vi "Read Data From run Files.vi"(0 "Rack":i8, 1 "Rack Position":i8, 2 ".run File Path":path=path "\\\\beco\\autoage/runs/pos", 3 "System Number":string) -> (4 "Serial Number":string, 5 "Unit Type":string, 6 "Customer":string, 7 "Nominal Frequency":string, 8 "Gate Time":string)   [LabVIEW 2021]
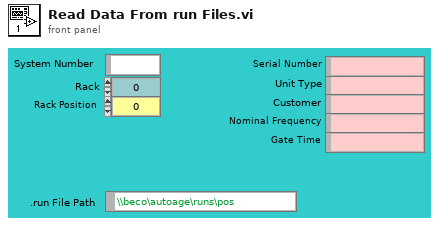
[diagram p1: front panel]
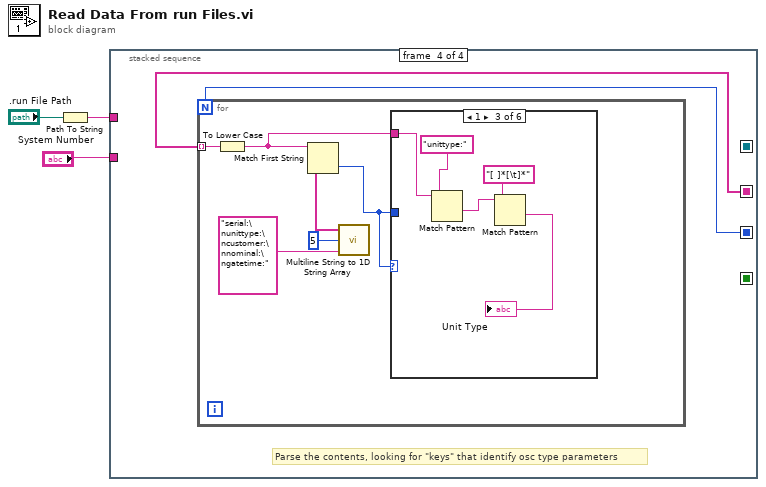
[diagram p0: block diagram]
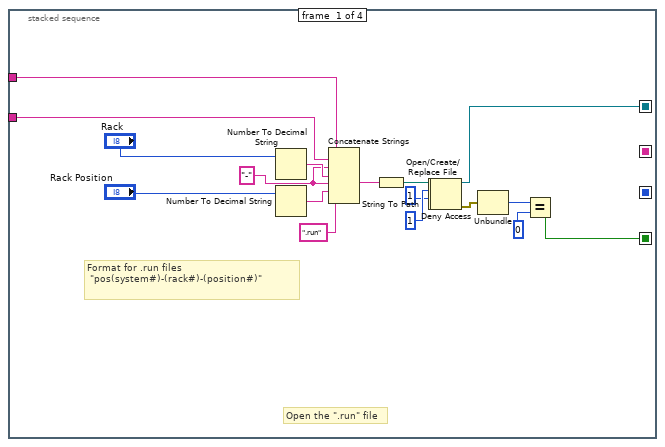
[diagram p2: hidden frame]
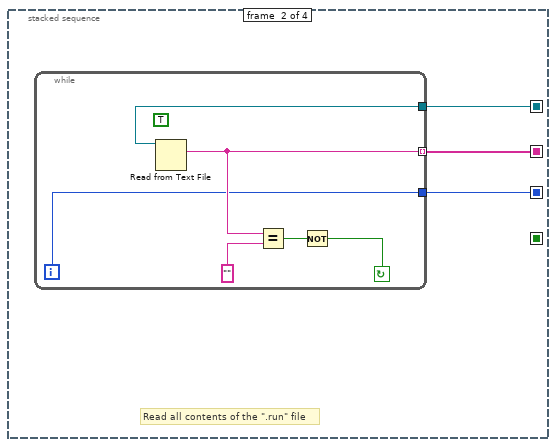
[diagram p3: hidden frame]
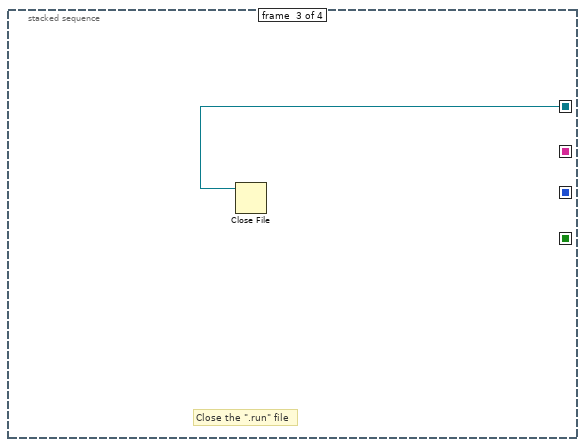
[diagram p4: hidden frame]
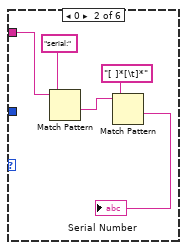
[diagram p6: hidden frame]
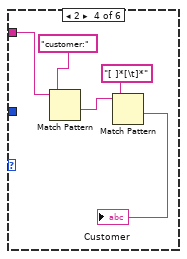
[diagram p7: hidden frame]
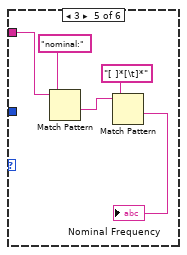
[diagram p8: hidden frame]
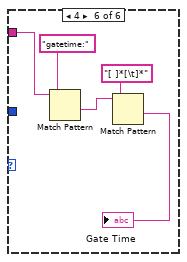
[diagram p9: hidden frame]
diagram:
  n1 = Path To String(path=".run File Path") -> (string=w1:string)
  n2 = stacked-sequence {
    seq-local: [w16 _ _ _] -> [_ w25 w32 _]
    seq-local: [w15 _ _ _] -> [_ _ _ _]
    seq-local: [_ w24 _ _] -> [_ _ _ w34]
    seq-local: [_ w23 _ _] -> [_ _ _ w33]
    tunnel: "System Number" -> [w7 _ _ _]
    tunnel: w1 -> [w6 _ _ _]
    frame #0 {
      w8 = "-"
      # "Format for .run files\n \"pos(system#)-(rack#)-(position#)\""
      # "Open the \".run\" file"
      n3 = Number To Decimal String(number="Rack") -> (decimal integer string=w14:string)  [unwired: 1 in]
      n4 = Number To Decimal String(number="Rack Position") -> (decimal integer string=w13:string)  [unwired: 1 in]
      n5 = Concatenate Strings(w6, w7, w8, w14, w8, w13, ".run") -> (w11:string)
      n6 = String To Path(string=w11) -> (path=w22:path)
      n7 = Open/Create/Replace File(file path (use dialog)=w22, access (0:read/write)=1) -> (refnum out=w4:refnum<file>, error out=w5:errorcluster)  [unwired: 4 in, 1 out]
      n8 = Deny Access(4:w5, 6:1, 7:w4) -> (0:w19:errorcluster, 3:w16:refnum<file>)
      n9 = Unbundle(w19) -> ("code"=w17:i32)  [unwired: 2 out]
      n10 = Equal?(x=w17, y=0) -> (x = y?=w15:bool)
    }
    frame #1 {
      # "Read all contents of the \".run\" file"
      n11 = while {
        tunnel: [w26] -> w23
        tunnel: [w27] -> w24 mode=indexing
        tunnel: w25 -> [w28]
        i -> [w26]
        stop <- w29 continue-if-true
        (unwired) TRUE
        n12 = Read from Text File(file (use dialog)=w28) -> (text=w27:string)  [unwired: 3 in, 3 out]
        n13 = Equal?(x=w27, y="") -> (x = y?=w30:bool)
        n14 = Not(x=w30) -> (.not. x?=w29:bool)
      }
    }
    frame #2 {
      # "Close the \".run\" file"
      n15 = Close File(refnum=w32) -> ()  [unwired: 1 in, 2 out]
    }
    frame #3 {
      # "Parse the contents, looking for \"keys\" that identify osc type parameters"
      n16 = for {
        N: w33 -> [_]
        tunnel: w34 -> [w38] mode=indexing
        n17 = To Lower Case(string=w38) -> (all lower case string=w35:string)
        n18 = call "Multiline String to 1D String Array.vi"("Multiline Input String"="serial:\nunittype:\ncustomer:\nnominal:\ngatetime:", "Number of Elements"=5) -> ("1D String Output Array"=w37:string[])
        n19 = Match First String(2:w37, 3:w35) -> (0:w36:i32)  [unwired: 1 out]
        n20 = case shown="1" w36 {
          tunnel: w35 -> [_ w45 w50 w55 w60 w65]
          tunnel: w36 -> [_ _ _ _ _ _]
          frame -1, Default {
          }
          frame 0 {
            n21 = Match Pattern(string=w45, regular expression="serial:") -> (after substring=w42:string)  [unwired: 1 in, 3 out]
            n22 = Match Pattern(string=w42, regular expression="[ ]*[\t]*") -> (after substring=→"Serial Number":string)  [unwired: 1 in, 3 out]
          }
          frame 1 {
            n23 = Match Pattern(string=w50, regular expression="unittype:") -> (after substring=w47:string)  [unwired: 1 in, 3 out]
            n24 = Match Pattern(string=w47, regular expression="[ ]*[\t]*") -> (after substring=→"Unit Type":string)  [unwired: 1 in, 3 out]
          }
          frame 2 {
            n25 = Match Pattern(string=w55, regular expression="customer:") -> (after substring=w52:string)  [unwired: 1 in, 3 out]
            n26 = Match Pattern(string=w52, regular expression="[ ]*[\t]*") -> (after substring=→"Customer":string)  [unwired: 1 in, 3 out]
          }
          frame 3 {
            n27 = Match Pattern(string=w60, regular expression="nominal:") -> (after substring=w57:string)  [unwired: 1 in, 3 out]
            n28 = Match Pattern(string=w57, regular expression="[ ]*[\t]*") -> (after substring=→"Nominal Frequency":string)  [unwired: 1 in, 3 out]
          }
          frame 4 {
            n29 = Match Pattern(string=w65, regular expression="gatetime:") -> (after substring=w62:string)  [unwired: 1 in, 3 out]
            n30 = Match Pattern(string=w62, regular expression="[ ]*[\t]*") -> (after substring=→"Gate Time":string)  [unwired: 1 in, 3 out]
          }
        }
      }
    }
  }
